vi "Read UID.vi"(11 "Queue Transport in":refnum<class "Queue Transport.lvclass">) -> (2 "UID":i32)   [LabVIEW 2020, in "jettl.lvlib" / "Queue Transport.lvlib" / "Queue Transport.lvclass"]
uses:
  Queue Transport.lvclass
  Queue Transport.lvclass/Queue Transport.ctl
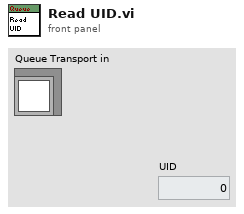
[diagram p1: front panel]
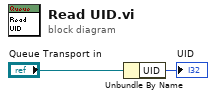
[diagram p0: block diagram]
diagram:
  n1 = Unbundle By Name("Queue Transport in") -> ("UID"=→"UID":i32)
